vi "CreatSendArray.vi"(0 "AngleSample":dbl[](array[numeric]), 4 "AxisForces":dbl[](array[numeric]), 6 "AccumulateSample":dbl[](array[numeric]), 7 "数组":dbl[](array[numeric]), 8 "DisplacementSample":dbl[](array[numeric]), 9 "ControlOutput":dbl[](array[numeric]), 10 "TorqueSampledata":dbl[](array[numeric]), 11 "Command":dbl[](array[numeric])) -> (3 "SendArray":dbl[](array[numeric]))   [LabVIEW 2020]
panel:
  out "AccumulateSample 2":dbl[](array[numeric])
  out "AngleSample 2":dbl[](array[numeric])
  out "DisplacementSample 2":dbl[](array[numeric])
  out "ControlOutput 2":dbl[](array[numeric])
  out "AxisForces 2":dbl[](array[numeric])
  out "TorqueSampledata 2":dbl[](array[numeric])
  out "Command 2":dbl[](array[numeric])
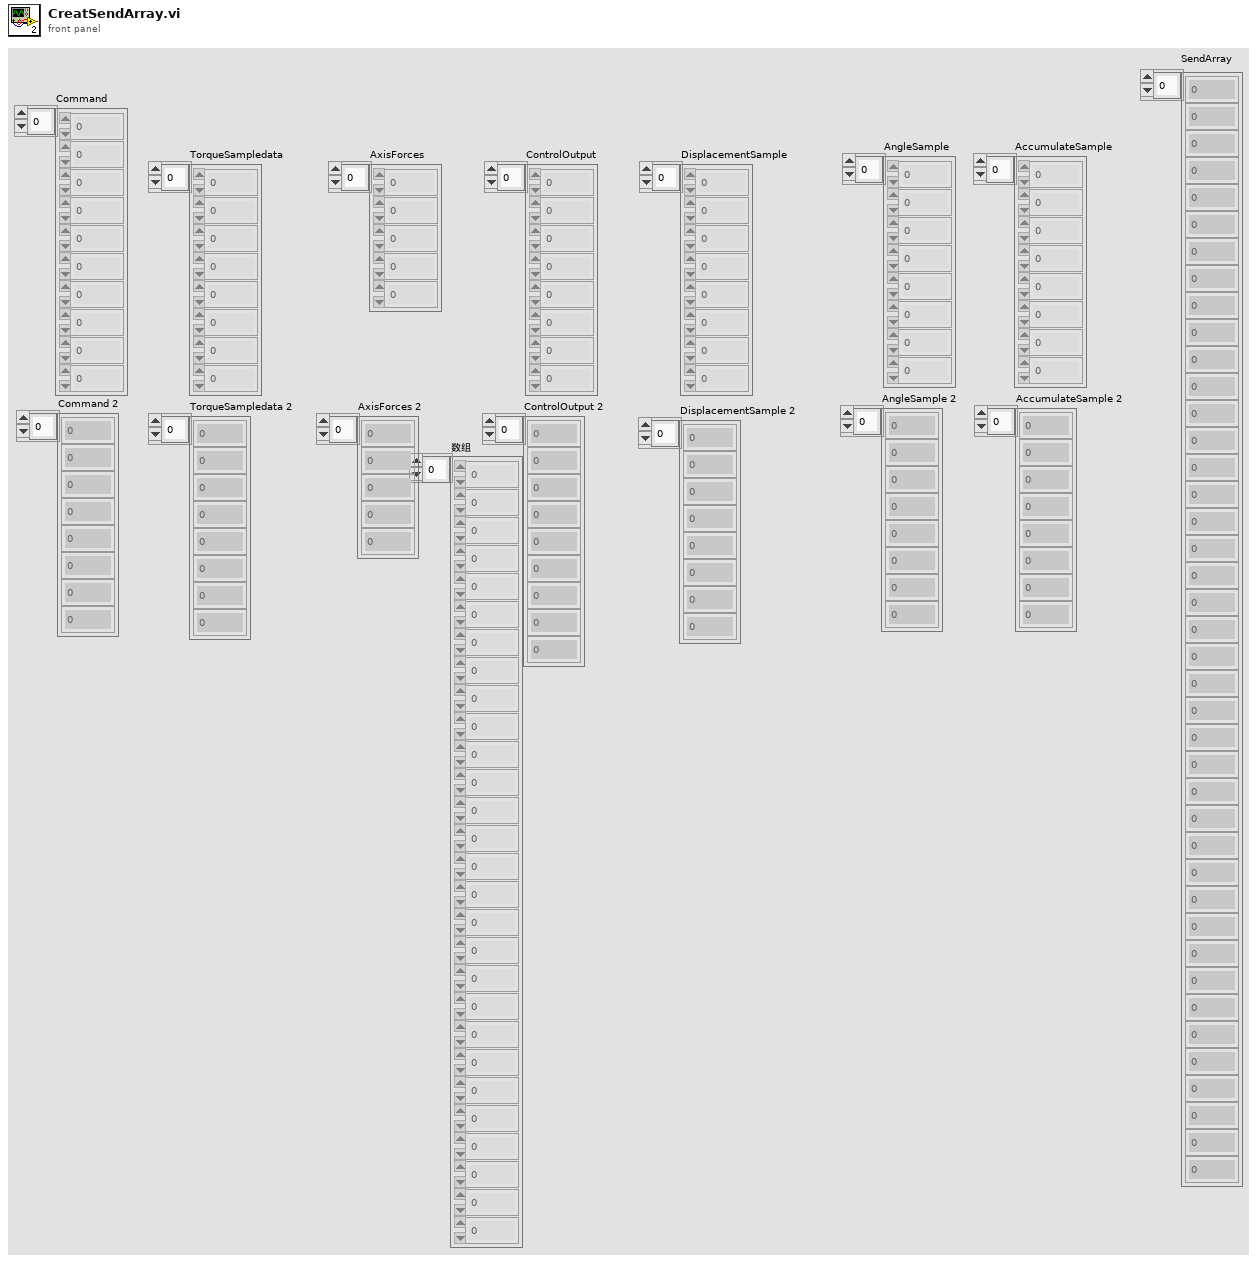
[diagram p1: front panel]
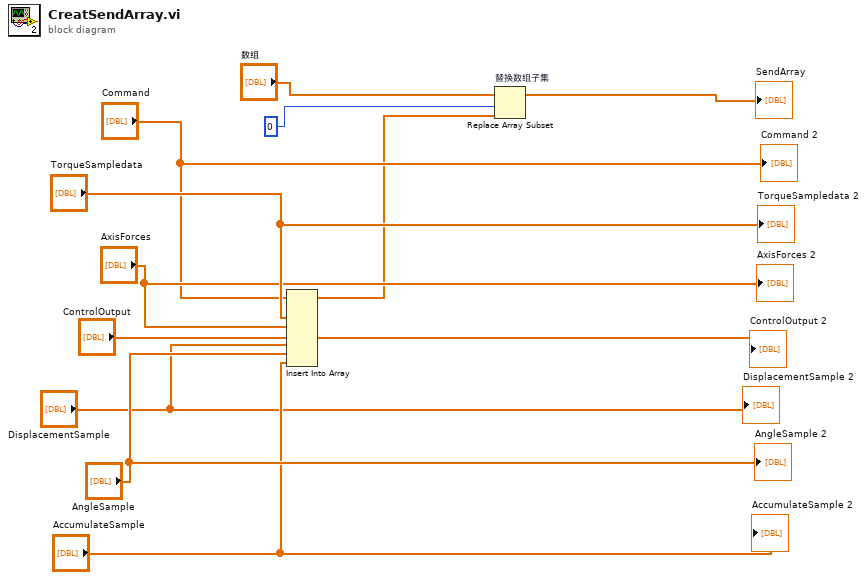
[diagram p0: block diagram]
diagram:
  n1 = Insert Into Array(array="Command", new element #1="TorqueSampledata", new element #2="AxisForces", new element #3="ControlOutput", new element #4="DisplacementSample", new element #5="AngleSample", new element #6="AccumulateSample") -> (w2:dbl[])  [unwired: 1 in]
  n2 = Replace Array Subset "替换数组子集"(array="数组", new element=w2, index=0 ("索引")) -> (→"SendArray":dbl[])
  "Command 2" <- "Command"
  "TorqueSampledata 2" <- "TorqueSampledata"
  "AxisForces 2" <- "AxisForces"
  "ControlOutput 2" <- "ControlOutput"
  "DisplacementSample 2" <- "DisplacementSample"
  "AngleSample 2" <- "AngleSample"
  "AccumulateSample 2" <- "AccumulateSample"
